vi "ex2.vi"() -> ()   [LabVIEW 2017]
uses:
  <vilib>/Utility/file.llb/Read Delimited Spreadsheet (string).vi
panel:
  out "Waveform Chart":dbl[][](graph)
  in  "Path to file":path
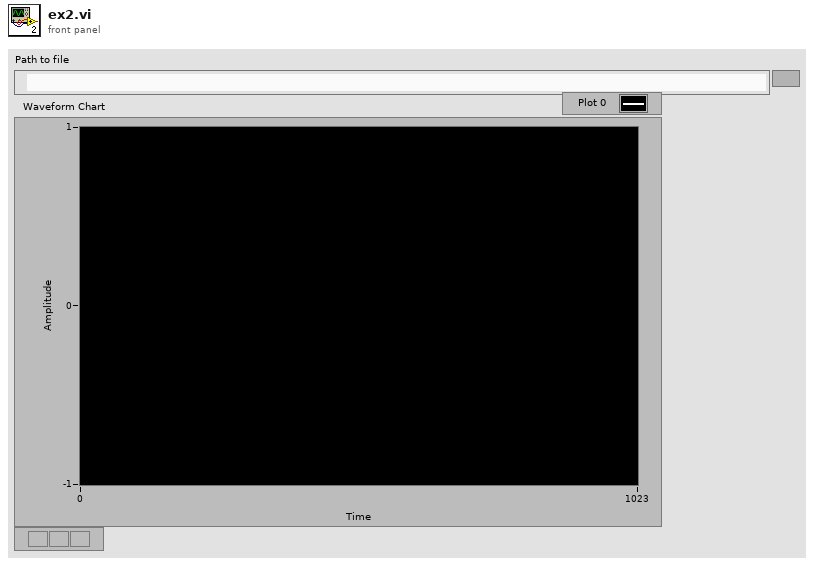
[diagram p1: front panel]
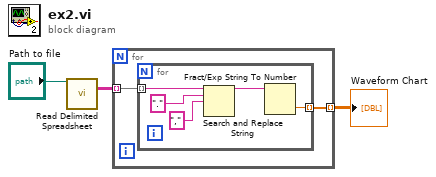
[diagram p0: block diagram]
diagram:
  n1 = call-poly <vilib>:"Read Delimited Spreadsheet.vi"("file path (dialog if empty)"="Path to file") -> ("all rows"=w2:string[][])  [unwired: 9 in, 5 out]
  n2 = for {
    tunnel: w2 -> [w5] mode=indexing
    tunnel: [w4] -> w1 mode=indexing
    n3 = for {
      tunnel: w5 -> [w10] mode=indexing
      tunnel: [w6] -> w4 mode=indexing
      n4 = Search and Replace String(input string=w10, search string=".", replace string="," ("replace string (\"\")")) -> (result string=w7:string)  [unwired: 5 in, 3 out]
      n5 = Fract/Exp String To Number(string=w7) -> (number=w6:dbl)  [unwired: 3 in, 1 out]
    }
  }
  "Waveform Chart" <- w1
